vi "Klaster_002_PH.vi"() -> ()   [LabVIEW 2021]
panel:
  out "cluster 2":T1={"Array"=[2020, 2020, 2020, 2020, 2020], "Boolean"=TRUE, "String"="Nowy napis"}
  in  "Cluster":T1={"Array"=[2020, 2020, 2020, 2020, 2020], "Boolean"=TRUE, "String"="pierwszy cluster"}
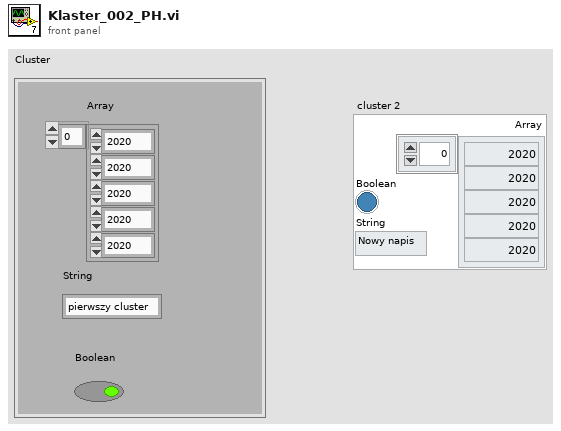
[diagram p1: front panel]
types:
  T1 = cluster{"Array":i16[], "Boolean":bool, "String":string}
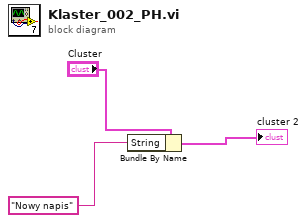
[diagram p0: block diagram]
diagram:
  n1 = Bundle By Name(cluster="Cluster", "String"="Nowy napis") -> (→"cluster 2":T1)
